vi "Read Keys.vi"(8 "error in (no error)":errorcluster, 11 "Configuration in":refnum<class "Configuration.lvclass">) -> (0 "error out":errorcluster, 2 "Keys":string[](array[string]), 3 "Configuration out":refnum<class "Configuration.lvclass">)   [LabVIEW 2023, in "Configuration.lvlib" / "Configuration.lvclass"]
uses:
  Library/Configuration.lvclass
  Library/Configuration.lvclass/Configuration.ctl
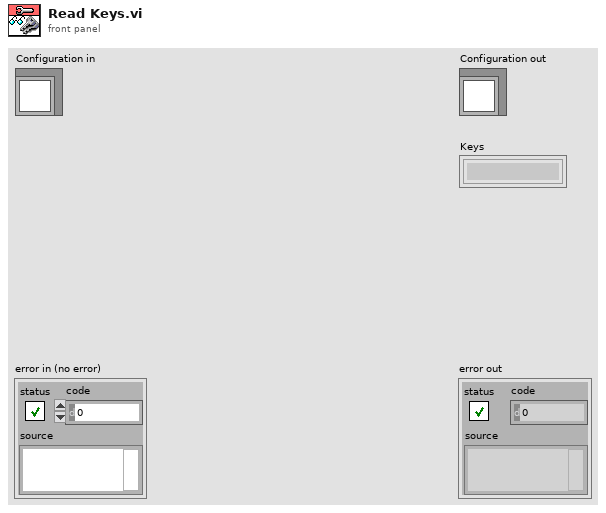
[diagram p1: front panel]
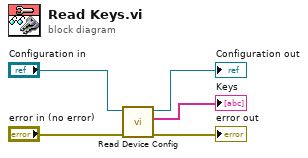
[diagram p0: block diagram]
diagram:
  n1 = call "Read Device Config.vi"("error in (no error)"="error in (no error)", "Configuration in"="Configuration in") -> ("error out"=→"error out":errorcluster, "Keys"=→"Keys":string[], "Configuration out"=→"Configuration out":refnum<class "Configuration.lvclass">)  [unwired: 6 in, 1 out]
